vi "equ_solver.vi"(2 "theta":dbl[](array[numeric]), 3 "Coordination":dbl[][](array[numeric])) -> (0 "now Y":dbl, 1 "now X":dbl)   [LabVIEW 2017]
uses:
  <vilib>/gmath/zero.llb/nD Nonlinear System Single Solution (Formula).vi
  <vilib>/express/express arith-compare/Formula/XNode/ExpressFormulaBlockNode.xnode
  <vilib>/gmath/NI_Gmath.lvlib
panel:
  out "Zeroes":dbl[](array[numeric]) format="%0.2f"
  out "appended array":string[](array[string])
  out "error(0 = no error)":i32
  out "ticks (ms)":u32
  in  "X":string[](array[string])=["x", "y"]
  in  "Initial guess":dbl[](array[numeric])=[-1.0, 2.0]
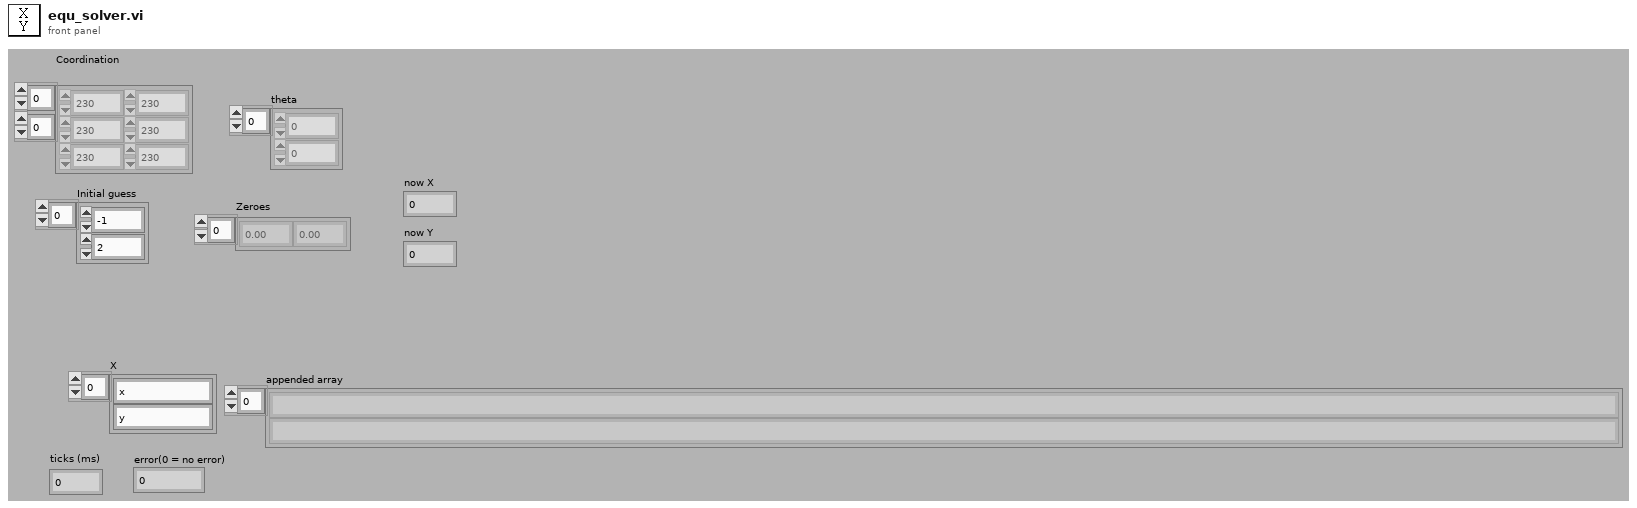
[diagram p1: front panel]
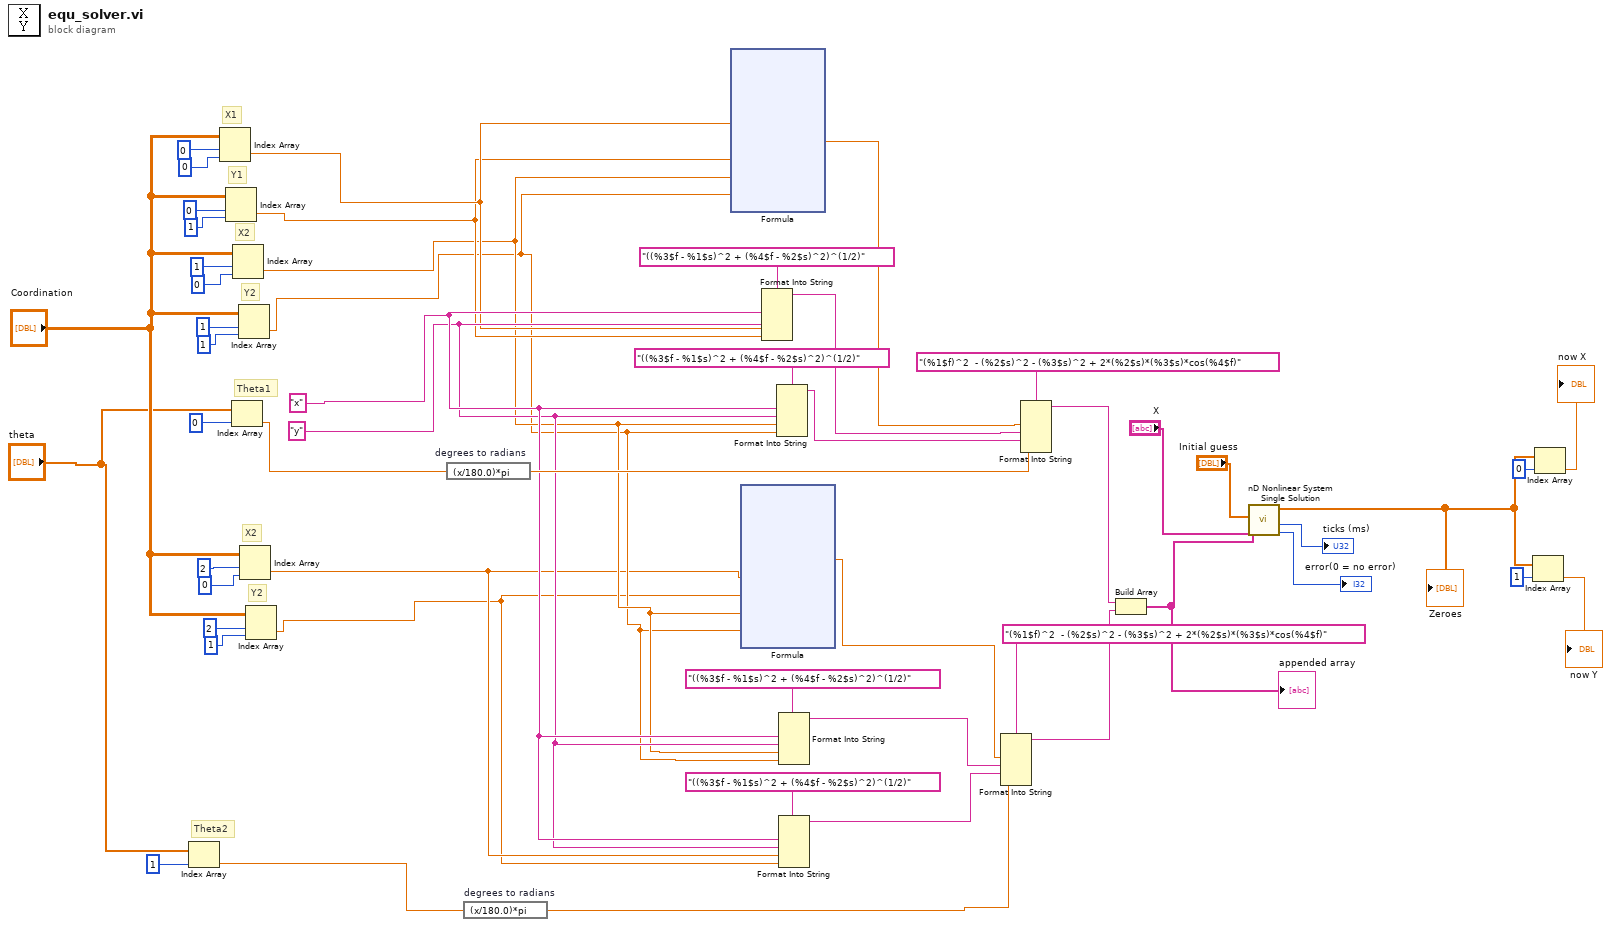
[diagram p0: block diagram]
diagram:
  w36 = "y" ("input 2")
  w37 = "x" ("input 1")
  # "Theta2"
  # "Theta1"
  # "Y2"
  # "X2"
  # "Y2"
  # "X2"
  # "Y1"
  # "X1"
  n1 = Index Array(array="theta", index=1) -> (element=w7:dbl)
  n2 = Index Array(array="Coordination", index (row)=0 ("index"), index (col)=0 ("disabled index (col)")) -> (element=w28:dbl)
  n3 = Index Array(array="Coordination", index (row)=0 ("index"), index (col)=1 ("disabled index (col)")) -> (element=w24:dbl)
  n4 = Index Array(array="theta", index=0) -> (element=w6:dbl)
  n5 = Index Array(array="Coordination", index (row)=1 ("index"), index (col)=0 ("disabled index (col)")) -> (element=w19:dbl)
  n6 = Index Array(array="Coordination", index (row)=1 ("index"), index (col)=1 ("disabled index (col)")) -> (element=w18:dbl)
  n7 = Index Array(array="Coordination", index (row)=2 ("index"), index (col)=0 ("disabled index (col)")) -> (element=w12:dbl)
  n8 = Index Array(array="Coordination", index (row)=2 ("index"), index (col)=1 ("disabled index (col)")) -> (element=w11:dbl)
  n9 = expression code="(x/180.0)*pi" "degrees to radians"(w6) -> (w39:dbl)
  n10 = expression code="(x/180.0)*pi" "degrees to radians"(w7) -> (w38:dbl)
  n11 = xnode "Formula"("X1"=w28, "Y1"=w24, "X2"=w19, "Y2"=w18) -> ("Result"=w43:dbl)  [unwired: 1 in, 1 out]
  n12 = xnode "Formula"("X3"=w12, "Y3"=w11, "X2"=w19, "Y2"=w18) -> ("Result"=w45:dbl)  [unwired: 1 in, 1 out]
  n13 = Format Into String(format string="((%3$f - %1$s)^2 + (%4$f - %2$s)^2)^(1/2)", w37, w36, w28, w24) -> (resulting string=w42:string)  [unwired: 2 in, 1 out]
  n14 = Format Into String(format string="((%3$f - %1$s)^2 + (%4$f - %2$s)^2)^(1/2)", w37, w36, w19, w18) -> (resulting string=w41:string)  [unwired: 2 in, 1 out]
  n15 = Format Into String(format string="((%3$f - %1$s)^2 + (%4$f - %2$s)^2)^(1/2)", w37, w36, w19, w18) -> (resulting string=w46:string)  [unwired: 2 in, 1 out]
  n16 = Format Into String(format string="((%3$f - %1$s)^2 + (%4$f - %2$s)^2)^(1/2)", w37, w36, w12, w11) -> (resulting string=w47:string)  [unwired: 2 in, 1 out]
  n17 = Format Into String(format string="(%1$f)^2  - (%2$s)^2 - (%3$s)^2 + 2*(%2$s)*(%3$s)*cos(%4$f)", w45, w46, w47, w38) -> (resulting string=w35:string)  [unwired: 2 in, 1 out]
  n18 = Format Into String(format string="(%1$f)^2  - (%2$s)^2 - (%3$s)^2 + 2*(%2$s)*(%3$s)*cos(%4$f)", w43, w42, w41, w39) -> (resulting string=w40:string)  [unwired: 2 in, 1 out]
  n19 = Build Array(w40, w35) -> (w30:string[])
  "appended array" <- w30
  n20 = call-poly <vilib>:"nD Nonlinear System Single Solution.vi"("F(X)"=w30, "X"="X", "Start"="Initial guess") -> ("error"=→"error(0 = no error)":i32, "ticks"=→"ticks (ms)":u32, "Zeroes"=w1:dbl[])  [unwired: 5 in, 1 out]
  "Zeroes" <- w1
  n21 = Index Array(array=w1, index=1) -> (element=→"now Y":dbl)
  n22 = Index Array(array=w1, index=0) -> (element=→"now X":dbl)
